vi "rvc Control Mixer.vi"(8 "Tau":dbl, 9 "Tau yaw":dbl, 10 "Tau roll":dbl, 11 "Tau Pitch":dbl) -> (0 "omega 4":dbl, 1 "omega 3":dbl, 2 "omega 2":dbl, 3 "omega 1":dbl)   [LabVIEW 2013]
uses:
  <vilib>/imath/engines/lvmath2/RunTimeEngine/ErrorHandling/NIMS_Finalize Error.vi
  <vilib>/imath/engines/lvmath2/RunTimeEngine/NodeEndStatement/NIMS_NodeEndStatement_Output.vi
  <instcachedir>/0/NIMS_NodeEndStatement_Output_53EC0D466D134D7ABD903AC30B43404B.lvgen/NIMS_NodeEndStatement_Output_53EC0D466D134D7ABD903AC30B43404B_002.vi
  <vilib>/imath/engines/lvmath2/RunTimeEngine/BuiltInFunctions/inv/NIMS_inv(GM).vi
  <instcachedir>/0/NIMS_inv(GM)_A6DF8FE880224208AACFE4CF9F659502.lvgen/NIMS_inv(GM)_A6DF8FE880224208AACFE4CF9F659502_000.vi
  <vilib>/imath/engines/lvmath2/RunTimeEngine/ErrorHandling/NIMS_Error From Error Code.vi
  <vilib>/imath/engines/lvmath2/RunTimeEngine/ArithmeticOperatorToken/NIMS_ArithmeticOperator_multmx(M,CV).vi
  <instcachedir>/0/NIMS_ArithmeticOperator_multmx(M,CV)_90351521EAFF49D48526FCD9D8E924F7.lvgen/NIMS_ArithmeticOperator_multmx(M,CV)_90351521EAFF49D48526FCD9D8E924F7_000.vi
  <vilib>/imathl/engines/lvmath/Functions/Error Handling/Create Error.vi
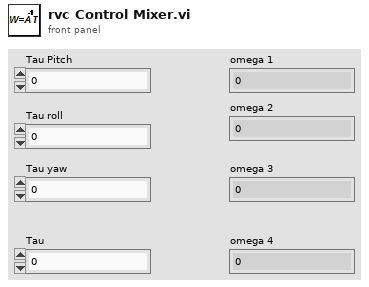
[diagram p1: front panel]
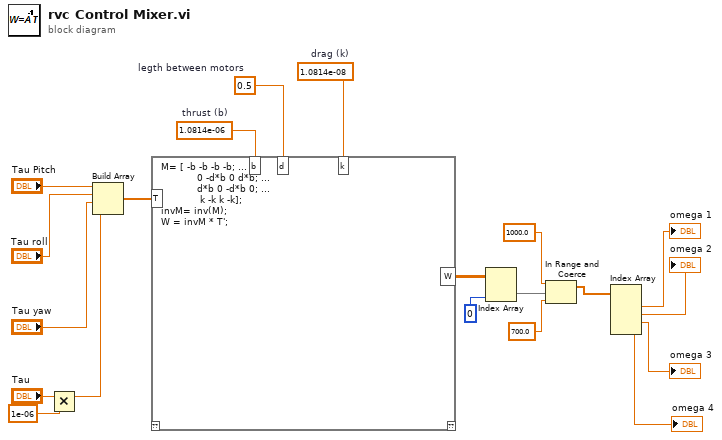
[diagram p0: block diagram]
diagram:
  w13 = 1.0814e-08  # drag (k)
  w14 = 0.5  # legth between motors
  w15 = 1.0814e-06  # thrust (b)
  n1 = Multiply(x="Tau", y=1e-06) -> (x*y=w6:dbl)
  n2 = Build Array("Tau Pitch", "Tau roll", "Tau yaw", w6) -> (w19:dbl[])
  n3 = mathscript code="M= [ -b -b -b -b; ...\n            0 -d*b 0 d*b; ...\n            d*b 0 -d*b 0; ...\n             k -k k -k];\ninvM= inv(M);\nW = invM * T';"("T"=w19, "b"=w15, "d"=w14, "k"=w13) -> ("W"=w12:dbl[][])  [unwired: 1 in, 1 out]
  n4 = Index Array(array=w12, index (col)=0 ("disabled index (col)")) -> (element=w4:dbl[])  [unwired: 1 in]
  n5 = In Range and Coerce(upper limit=1000.0, x=w4, lower limit=700.0) -> (coerced(x)=w1:dbl[])  [unwired: 1 out]
  n6 = Index Array(array=w1) -> (element #1=→"omega 1":dbl, element #2=→"omega 2":dbl, element #3=→"omega 3":dbl, element #4=→"omega 4":dbl)  [unwired: 4 in]
